vi "Execute.vi"(8 "error in":errorcluster, 11 "Tasks in":refnum<class "Tasks.lvclass">) -> (0 "error out":errorcluster, 1 "Next Step?":bool, 2 "MSG":string, 3 "Tasks out":refnum<class "Tasks.lvclass">)   [LabVIEW 2012, in "Tasks.lvclass"]
uses:
  Tasks.lvclass
  <vilib>/Utility/miscctls.llb/LVDateTimeRec.ctl
  Tasks.lvclass/Tasks.ctl
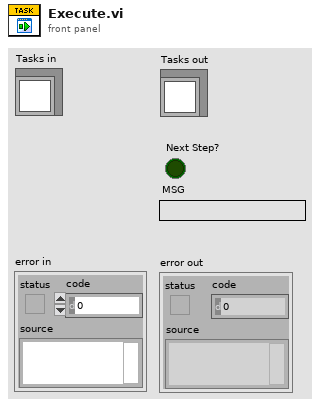
[diagram p1: front panel]
types:
  T1 = typedef "LVDateTimeRec.ctl" = cluster{"fractional second":dbl, "second":i32, "minute":i32, "hour":i32, "day of month":i32, "month":i32, "year":i32, "day of week":i32, "day of year":i32, "DST":i32}
  T2 = typedef "Mode Select.ctl" = enum8{"Off", "Stby", "Hold", "Run"}
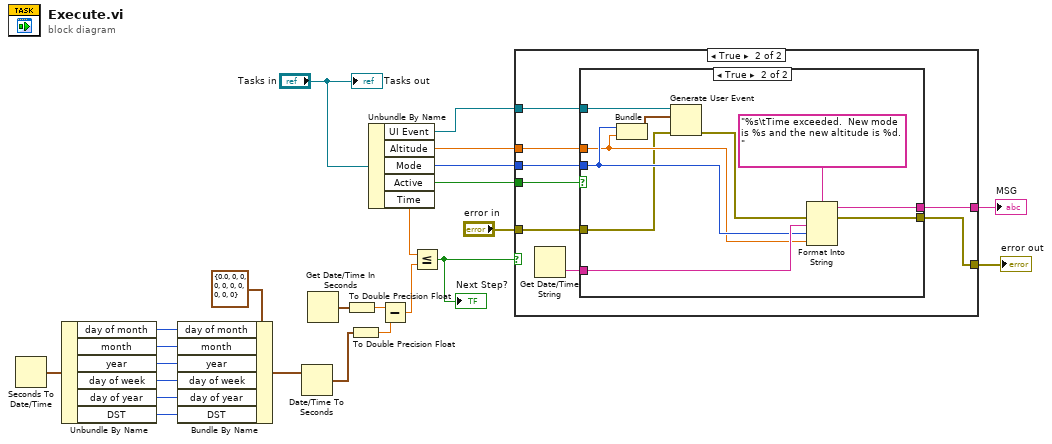
[diagram p0: block diagram]
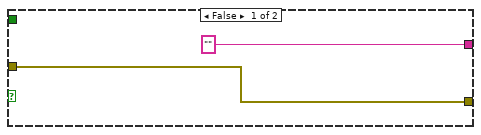
[diagram p2: hidden frame]
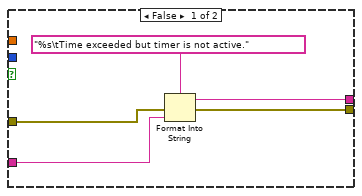
[diagram p3: hidden frame]
diagram:
  n1 = Seconds To Date/Time() -> (date time rec=w15:T1)  [unwired: 2 in]
  n2 = Unbundle By Name(w15) -> ("day of month"=w14:i32, "month"=w12:i32, "year"=w11:i32, "day of week"=w4:i32, "day of year"=w10:i32, "DST"=w9:i32)
  n3 = Bundle By Name(cluster=T1 {"fractional second"=0.0, "second"=0, "minute"=0, "hour"=0, "day of month"=0, "month"=0, "year"=0, "day of week"=0, "day of year"=0, "DST"=0} ("date time rec"), "day of month"=w14, "month"=w12, "year"=w11, "day of week"=w4, "day of year"=w10, "DST"=w9) -> (w13:T1)
  n4 = Date/Time To Seconds(2:w13) -> (0:w7:timestamp)  [unwired: 1 in]
  n5 = Get Date/Time In Seconds() -> (seconds since 1Jan1904=w8:timestamp)
  n6 = To Double Precision Float(number=w8) -> (double precision float=w5:dbl)
  n7 = To Double Precision Float(number=w7) -> (double precision float=w6:dbl)
  n8 = Unbundle By Name("Tasks in") -> ("UI Event"=w17:refnum<user-event>, "Altitude"=w21:sgl, "Mode"=w23:T2, "Active"=w1:bool, "Time"=w2:dbl)
  n9 = Subtract(x=w5, y=w6) -> (x-y=w3:dbl)
  n10 = Less Or Equal?(x=w2, y=w3) -> (x <= y?=w19:bool)
  "Next Step?" <- w19
  n11 = case shown="True" w19 {
    tunnel: w1 -> [_ w33]
    tunnel: w23 -> [_ w32]
    tunnel: ["" w31] -> w22
    tunnel: w21 -> [_ w30]
    tunnel: [w26 w29] -> w20
    tunnel: "error in" -> [w26 w28]
    tunnel: w17 -> [_ w27]
    frame False {
    }
    frame True {
      n12 = Get Date/Time String() -> (time string=w34:string)  [unwired: 3 in, 1 out]
      n13 = case shown="True" w33 {
        tunnel: w34 -> [w38 w48]
        tunnel: w32 -> [_ w45]
        tunnel: [w37 w47] -> w31
        tunnel: w30 -> [_ w44]
        tunnel: [w36 w46] -> w29
        tunnel: w28 -> [w35 w41]
        tunnel: w27 -> [_ w42]
        frame False {
          n14 = Format Into String(format string="%s\tTime exceeded but timer is not active.", error in=w35, w38) -> (resulting string=w37:string, error out=w36:errorcluster)  [unwired: 1 in]
        }
        frame True {
          n15 = Bundle("Mode"=w45, "Altitude"=w44) -> (w43:cluster{"Mode":T2, "Altitude":sgl})  [unwired: 1 in]
          n16 = Generate User Event(user event=w42, event data cluster=w43, error in=w41) -> (error out=w40:errorcluster)  [unwired: 1 out]
          n17 = Format Into String(format string="%s\tTime exceeded.  New mode is %s and the new altitude is %d.", error in=w40, w48, w45, w44) -> (resulting string=w47:string, error out=w46:errorcluster)  [unwired: 1 in]
        }
      }
    }
  }
  "error out" <- w20
  "MSG" <- w22
  "Tasks out" <- "Tasks in"
